vi "8HP_Standard_EnFlo_Specific.vi"(2 "Datalog file path (full)":path, 3 "COM port":refnum<visa-resource-name>, 4 "Log data stream":bool, 5 "Set data rate (Hz)":u8(ring)=14 items=["1", "2", "4", "5", "8", "10", "16", "20", "25", "32", "40", "50", "64", "80", "100", "125", "160", "200", "250", "320", "400", "500", "625", "800", "1000"], 6 "N samples":u32=1000, 7 "Command":T2="s") -> (0 "Error":errorcluster, 1 "All samples out":sgl[][](array[numeric]))   [LabVIEW 2020]
uses:
  ctls/8HP_Cmd (USB).ctl
  Globals/Meas_global.vi
panel:
  in  "Main":T1(tab)
  out "Serial number":sgl
  out "Subsystems ok":bool[](array[boolean])
  out "Pressure sensor values in range":bool[](array[boolean])
  out "Pressure sensor temperatures in range":bool[](array[boolean])
  out "Pressure sensor EEPROM checksums ok":bool[](array[boolean])
  out "P_raw_Azero":sgl[](array[numeric])
  out "n":u16
  out "Auto zero progBar":u16(slide) caption="Collecting samples, please maintain dP = 0" scale=0.0..1000.0
  in  "EEPROM array 2":u16[](array[numeric])
  in  "EEPROM array":sgl[](array[numeric])
  out "Chk ok":bool
  out "EEPROM Checksum":u8 format="%02x"
  out "received":bool
  out "Returned data rate (Hz)":u16
  out "sent":bool
  out "frm err":u32
  out "chk err":u32
  in  "Stop Data":bool
  out "Relative humidity (%)":sgl
  out "Env. sensor die temperature (deg C)":sgl
  out "External thermistor 0 temperature (deg C)":sgl
  out "Atmospheric pressure (mbar)":sgl
  out "Checksum ok":bool
  out "Gyration vector (deg / s)":sgl[](array[numeric])
  out "Acceleration vector (g)":sgl[](array[numeric])
  out "Pressures":sgl[][](graph)
  out "Stream enabled":bool
  out "External thermistor 1 temperature (deg C)":sgl
  # "Paul Nathan 07/2023"
  # "Output array order:\nP0 (Pa)\n  |\nP7 (Pa)\nT0 (deg C)\nT1 (deg C)\nP_atmos (mbar)\nT_env (deg C)\nRH (%)\nax (g)\nay (g)\naz (g)\nwx (deg / s)\nwy (deg / s)\nwz (deg / s)"
  # "Environmental sensor present"
  # "Inertial sensor present"
  # "Accelerometer self test pass"
  # "Gyroscope self test pass"
  # "External thermistor 0 value in range"
  # "External thermistor 1 value in range"
  # "MCU EEPROM checksum ok"
  # "Pressure sensor 0 value in range"
  # "Pressure sensor 1 value in range"
  # "Pressure sensor 2 value in range"
  # "Pressure sensor 3 value in range"
  # "Pressure sensor 4 value in range"
  # "Pressure sensor 5 value in range"
  # "Pressure sensor 6 value in range"
  # "Pressure sensor 7 value in range"
  # "Pressure sensor 0 temperature in range"
  # "Pressure sensor 1 temperature in range"
  # "Pressure sensor 2 temperature in range"
  # "Pressure sensor 3 temperature in range"
  # "Pressure sensor 4 temperature in range"
  # "Pressure sensor 5 temperature in range"
  # "Pressure sensor 6 temperature in range"
  # "Pressure sensor 7 temperature in range"
  # "Pressure sensor 0 EEPROM checksum okay"
  # "Pressure sensor 1 EEPROM checksum okay"
  # "Pressure sensor 2 EEPROM checksum okay"
  # "Pressure sensor 3 EEPROM checksum okay"
  # "Pressure sensor 4 EEPROM checksum okay"
  # "Pressure sensor 5 EEPROM checksum okay"
  # "Pressure sensor 6 EEPROM checksum okay"
  # "Pressure sensor 7 EEPROM checksum okay"
  # "of 1000"
  # "P0 raw auto-zero"
  # "P1 raw auto-zero"
  # "P2 raw auto-zero"
  # "P3 raw auto-zero"
  # "P4 raw auto-zero"
  # "P5 raw auto-zero"
  # "P6 raw auto-zero"
  # "P7 raw auto-zero"
  # "Power-up defaults"
  # "Data rate (Hz)"
  # "TTL streaming"
  # "USB streaming"
  # "TTL stream contains full data"
  # "Accelerometer range mode"
  # "Gyroscope range mode"
  # "IMU rate mode"
  # "P0 raw auto-zero"
  # "P1 raw auto-zero"
  # "P2 raw auto-zero"
  # "P3 raw auto-zero"
  # "P4 raw auto-zero"
  # "P5 raw auto-zero"
  # "P6 raw auto-zero"
  # "P7 raw auto-zero"
  # "Atmospheric pressure offset (Pa)"
  # "External thermistor 0 temperature offset (deg C)"
  # "External thermistor 1 temperature offset (deg C)"
  # "Serial number"
  # "Baud rate (bps)"
  # "Accelerometer vector magnitude scale factor"
  # "Gyroscope x component offset (deg / s)"
  # "Gyroscope y component offset (deg / s)"
  # "Gyroscope z component offset (deg / s)"
  # "w_x"
  # "w_y"
  # "w_z"
  # "a_x"
  # "a_y"
  # "a_z"
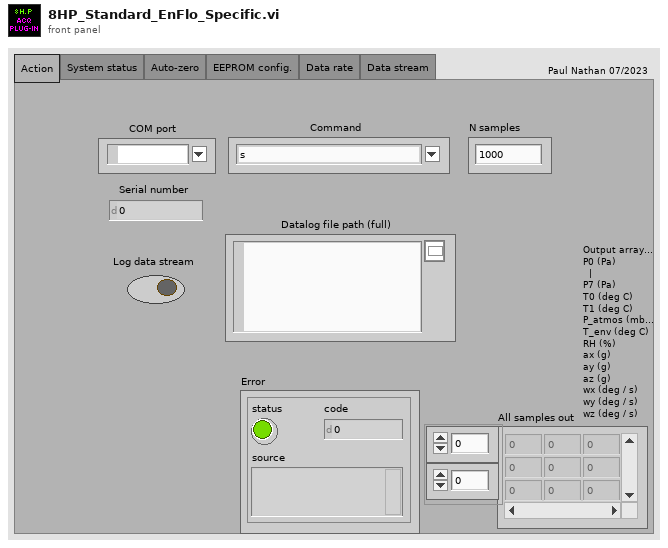
[diagram p1: front panel]
types:
  T1 = enum32{"Action", "System status", "Auto-zero", "EEPROM config.", "Data rate", "Data stream"}
  T2 = typedef "8HP_Cmd (USB).ctl" = string
  T3 = enum16{"open", "replace", "create", "open or create", "replace or create", "replace or create with confirmation"}
  T4 = typedef "Rendezvous RefNum" = refnum<k1>
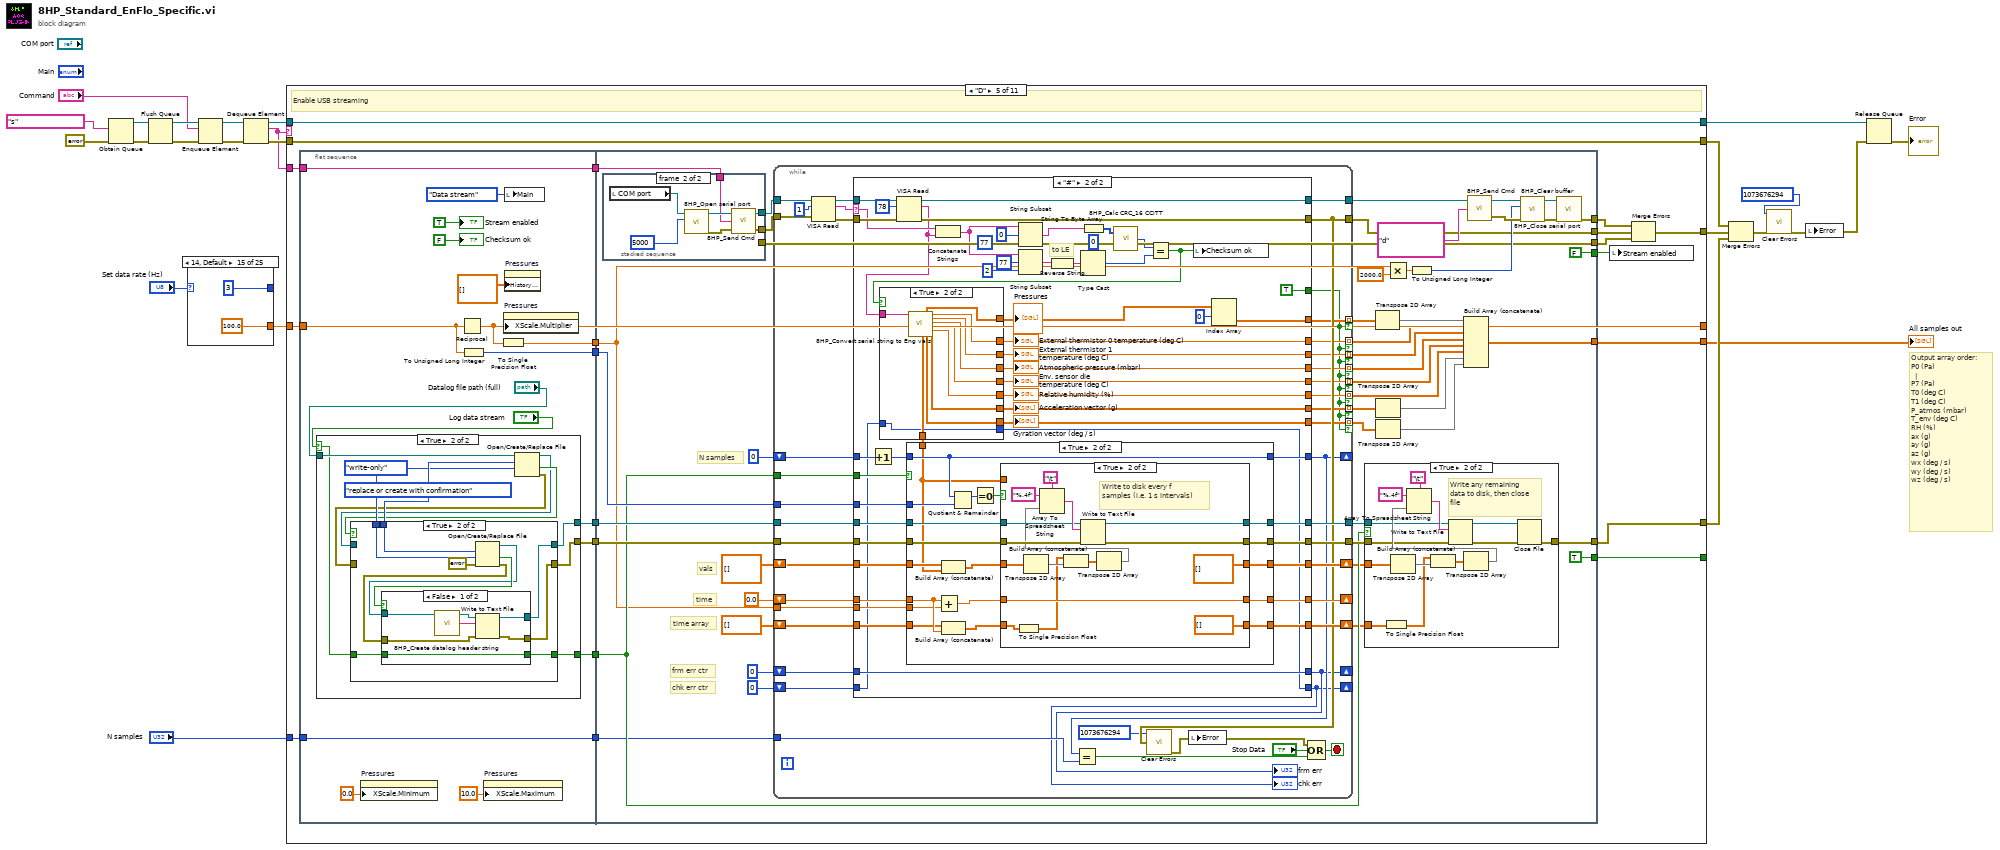
[diagram p0: block diagram]
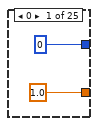
[diagram p2: hidden frame]
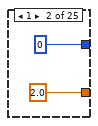
[diagram p3: hidden frame]
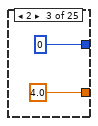
[diagram p4: hidden frame]
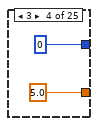
[diagram p5: hidden frame]
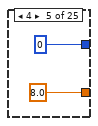
[diagram p6: hidden frame]
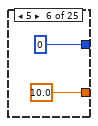
[diagram p7: hidden frame]
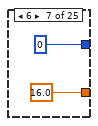
[diagram p8: hidden frame]
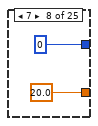
[diagram p9: hidden frame]
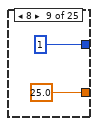
[diagram p10: hidden frame]
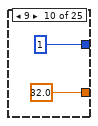
[diagram p11: hidden frame]
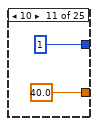
[diagram p12: hidden frame]
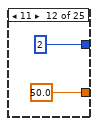
[diagram p13: hidden frame]
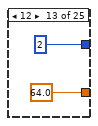
[diagram p14: hidden frame]
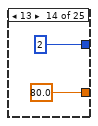
[diagram p15: hidden frame]
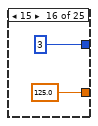
[diagram p16: hidden frame]
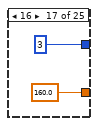
[diagram p17: hidden frame]
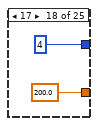
[diagram p18: hidden frame]
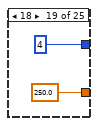
[diagram p19: hidden frame]
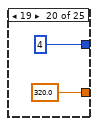
[diagram p20: hidden frame]
diagram:
  # "Output array order:\nP0 (Pa)\n  |\nP7 (Pa)\nT0 (deg C)\nT1 (deg C)\nP_atmos (mbar)\nT_env (deg C)\nRH (%)\nax (g)\nay (g)\naz (g)\nwx (deg / s)\nwy (deg / s)\nwz (deg / s)"
  n1 = Obtain Queue(element data type=T2 "s" ("Combo Box"), error in (no error)=errorcluster {"status"=FALSE, "code"=0, "source"=""}) -> (queue out=w22:refnum<queue>, error out=w23:errorcluster)  [unwired: 3 in, 1 out]
  n2 = Flush Queue(queue=w22, error in (no error)=w23) -> (queue out=w17:refnum<queue>, error out=w16:errorcluster)  [unwired: 1 out]
  n3 = case shown="14, Default" "Set data rate (Hz)" {
    tunnel: [1.0 2.0 4.0 5.0 8.0 10.0 16.0 20.0 25.0 32.0 40.0 50.0 64.0 80.0 100.0 125.0 160.0 200.0 250.0 320.0 400.0 500.0 625.0 800.0 1000.0] -> w4
    tunnel: [u8 0 u8 0 u8 0 u8 0 u8 0 u8 0 u8 0 u8 0 u8 1 u8 1 u8 1 u8 2 u8 2 u8 2 u8 3 u8 3 u8 3 u8 4 u8 4 u8 4 u8 5 u8 5 u8 6 u8 6 u8 6] -> _
    frame 0 {
    }
    frame 1 {
    }
    frame 2 {
    }
    frame 3 {
    }
    frame 4 {
    }
    frame 5 {
    }
    frame 6 {
    }
    frame 7 {
    }
    frame 8 {
    }
    frame 9 {
    }
    frame 10 {
    }
    frame 11 {
    }
    frame 12 {
    }
    frame 13 {
    }
    frame 14, Default {
    }
    frame 15 {
    }
    frame 16 {
    }
    frame 17 {
    }
    frame 18 {
    }
    frame 19 {
    }
    frame 20 {
    }
    frame 21 {
    }
    frame 22 {
    }
    frame 23 {
    }
    frame 24 {
    }
  }
  n4 = Enqueue Element(queue=w17, element="Command", error in (no error)=w16) -> (queue out=w19:refnum<queue>, error out=w18:errorcluster)  [unwired: 1 in, 1 out]
  n5 = Dequeue Element(queue=w19, error in (no error)=w18) -> (queue out=w14:refnum<queue>, element=w12:T2, error out=w13:errorcluster)  [unwired: 1 in, 1 out]
  n6 = case shown="\"D\"" w12 {
    tunnel: [w81 w122 w161 w237 w315 w618 w644 w727 w767 FALSE FALSE] -> _
    tunnel: w14 -> [w80 w121 w160 w236 w314 w620 w646 w729 w766 w791 w796]
    tunnel: [w80 w121 w160 w236 w314 w620 w646 w729 w766 w791 w796] -> w6
    tunnel: w13 -> [w79 w120 w159 w235 w313 w619 w647 w730 w765 w790 w795]
    tunnel: [w79 w120 w159 w235 w313 w619 w647 w730 w765 w790 w795] -> w11
    tunnel: w12 -> [w78 w119 w158 w234 w312 w622 w652 w735 w764 _ _]
    tunnel: [w76 w117 w156 w231 w298 w621 w645 w728 w762 errorcluster {"status"=FALSE, "code"=0, "source"=""} ("Error out") errorcluster {"status"=FALSE, "code"=0, "source"=""} ("Error out")] -> w10
    tunnel: [_ _ _ _ w310 _ _ _ _ _ _] -> w9
    tunnel: w4 -> [w75 w116 w155 w230 w303 w616 _ _ w761 w787 w792]
    tunnel: [w75 w116 w155 w230 w303 w616 w648 w731 w761 w787 w792] -> _
    tunnel: [_ _ _ _ w302 _ _ _ _ _ _] -> w2
    tunnel: "N samples" -> [_ _ _ _ w296 _ _ _ _ _ _]
    frame "S", "s" {
      # "Perform self-test and retrieve status bytes, Retrieve status bytes"
      n7 = flat-sequence {
        tunnel: w78 -> [w84]
        tunnel: [w84] -> w77
        tunnel: [TRUE] -> w81
        tunnel: w77 -> [w90]
        tunnel: [w85] -> w76
        frame #0 {
          w83 = bool[] [] ("Pressure sensor EEPROM checksums ok")
          n8 = local write "Main"(T1."System status" ("Main")) -> ()
          "Pressure sensor EEPROM checksums ok" <- w83
          "Pressure sensor temperatures in range" <- w83
          "Pressure sensor values in range" <- w83
          "Subsystems ok" <- w83
        }
        frame #1 {
          w95 = 1 ("length (rest)")
          w103 = u8 0 ("byte count")
          n9 = local read "COM port"() -> (w91:refnum<visa-resource-name>)
          n10 = call "8HP_Open serial port.vi"("timeout (ms)"=u32 5000, "VISA resource name"=w91) -> ("Error out"=w113:errorcluster, "VISA resource name out"=w114:refnum<visa-resource-name>)  [unwired: 8 in]
          n11 = call "8HP_Send Cmd.vi"("Error In"=w113, "Operation"=w90, "Port"=w114) -> ("Error Out"=w111:errorcluster, "Port out"=w112:refnum<visa-resource-name>)  [unwired: 1 in]
          n12 = VISA Read(VISA resource name=w112, byte count=u32 4, error in (no error)=w111) -> (VISA resource name out=w109:refnum<visa-resource-name>, read buffer=w98:string, error out=w108:errorcluster)  [unwired: 1 out]
          n13 = call "8HP_Close serial port.vi"("Error in"=w108, "VISA resource name"=w109) -> ("Error out"=w85:errorcluster)  [unwired: 9 in]
          n14 = String Subset(string=w98, offset (0)=0, length (rest)=w95) -> (substring=w107:string)
          n15 = String Subset(string=w98, offset (0)=1, length (rest)=w95) -> (substring=w106:string)
          n16 = String Subset(string=w98, offset (0)=2 ("length (rest)"), length (rest)=w95) -> (substring=w105:string)
          n17 = String Subset(string=w98, offset (0)=3, length (rest)=w95) -> (substring=w104:string)
          n18 = Type Cast(type=w103, x=w107) -> (*(type *) &x=w102:u8)
          n19 = Type Cast(type=w103, x=w106) -> (*(type *) &x=w101:u8)
          n20 = Type Cast(type=w103, x=w105) -> (*(type *) &x=w100:u8)
          n21 = Type Cast(type=w103, x=w104) -> (*(type *) &x=w99:u8)
          n22 = Number To Boolean Array(number=w102) -> (Boolean array=w89:bool[])
          n23 = Number To Boolean Array(number=w101) -> (Boolean array=w88:bool[])
          n24 = Number To Boolean Array(number=w100) -> (Boolean array=w87:bool[])
          n25 = Number To Boolean Array(number=w99) -> (Boolean array=w86:bool[])
          n26 = local write "Pressure sensor EEPROM checksums ok"(w89) -> ()
          n27 = local write "Pressure sensor temperatures in range"(w88) -> ()
          n28 = local write "Pressure sensor values in range"(w87) -> ()
          n29 = local write "Subsystems ok"(w86) -> ()
        }
      }
    }
    frame "Z", "z" {
      # "Perform permanent auto-zero (write values to EEPROM), Perform temporary auto-zero"
      n30 = flat-sequence {
        tunnel: w119 -> [w126]
        tunnel: [w126] -> w118
        tunnel: [TRUE] -> w122
        tunnel: w118 -> [w133]
        tunnel: [w129] -> w117
        frame #0 {
          n31 = local write "Main"(T1."Auto-zero" ("Main")) -> ()
          "P_raw_Azero" <- sgl[] [] ("P_raw_Azero")
          "Auto zero progBar" <- u16 0 ("Collecting samples, please maintain dP = 0")
        }
        frame #1 {
          n32 = local read "COM port"() -> (w134:refnum<visa-resource-name>)
          n33 = call "8HP_Open serial port.vi"("timeout (ms)"=u32 16000, "VISA resource name"=w134) -> ("Error out"=w141:errorcluster, "VISA resource name out"=w142:refnum<visa-resource-name>)  [unwired: 8 in]
          n34 = call "8HP_Send Cmd.vi"("Error In"=w141, "Operation"=w133, "Port"=w142) -> ("Error Out"=w139:errorcluster, "Port out"=w140:refnum<visa-resource-name>)  [unwired: 1 in]
          n35 = VISA Read(VISA resource name=w140, byte count=u32 32, error in (no error)=w139) -> (VISA resource name out=w137:refnum<visa-resource-name>, read buffer=w130:string, error out=w136:errorcluster)  [unwired: 1 out]
          n36 = for {
            N: 1000 -> [_]
            shift-right: [w144] -> _
            shift-left: u16 0 -> [w145]
            n37 = Increment(x=w145) -> (x+1=w144:u16)
            "n" <- w144
            n38 = Wait (ms)(milliseconds to wait=u32 10) -> ()  [unwired: 1 out]
            n39 = local write "Auto zero progBar"(w144) -> ()
          }
          n40 = for {
            N: 8 -> [_]
            tunnel: [w148] -> w132 mode=indexing
            tunnel: w130 -> [w147]
            i -> [w154]
            w152 = 4 ("x")
            # "to BE"
            n41 = Multiply(x=w152, y=w154) -> (x*y=w153:i32)
            n42 = String Subset(string=w147, offset (0)=w153, length (rest)=w152) -> (substring=w151:string)
            n43 = Reverse String(1:w151) -> (0:w150:string)
            n44 = Type Cast(type=sgl 0.0 ("byte count"), x=w150) -> (*(type *) &x=w148:sgl)
          }
          n45 = call "8HP_Close serial port.vi"("Error in"=w136, "VISA resource name"=w137) -> ("Error out"=w129:errorcluster)  [unwired: 9 in]
          n46 = local write "P_raw_Azero"(w132) -> ()
        }
      }
    }
    frame "R" {
      # "Read all EEPROM values"
      n47 = flat-sequence {
        tunnel: w158 -> [w165]
        tunnel: [w165] -> w157
        tunnel: [TRUE] -> w161
        tunnel: w157 -> [w200]
        tunnel: [w189] -> w156
        frame #0 {
          n48 = local write "EEPROM array"(sgl[] [] ("EEPROM array")) -> ()
          n49 = local write "EEPROM array 2"(u16[] [] ("EEPROM array 2")) -> ()
          n50 = local write "Main"(T1."EEPROM config." ("Main")) -> ()
        }
        frame #1 {
          # "to BE"
          n51 = local read "COM port"() -> (w201:refnum<visa-resource-name>)
          n52 = call "8HP_Open serial port.vi"("timeout (ms)"=u32 5000, "VISA resource name"=w201) -> ("Error out"=w208:errorcluster, "VISA resource name out"=w209:refnum<visa-resource-name>)  [unwired: 8 in]
          n53 = call "8HP_Send Cmd.vi"("Error In"=w208, "Operation"=w200, "Port"=w209) -> ("Error Out"=w206:errorcluster, "Port out"=w207:refnum<visa-resource-name>)  [unwired: 1 in]
          n54 = VISA Read(VISA resource name=w207, byte count=u32 78, error in (no error)=w206) -> (VISA resource name out=w204:refnum<visa-resource-name>, read buffer=w172:string, error out=w203:errorcluster)  [unwired: 1 out]
          n55 = String To Byte Array(string=w172) -> (unsigned byte array=w192:u8[])
          n56 = call "8HP_Close serial port.vi"("Error in"=w203, "VISA resource name"=w204) -> ("Error out"=w189:errorcluster)  [unwired: 9 in]
          n57 = String Subset(string=w172, offset (0)=0, length (rest)=56 ("length (rest)")) -> (substring=w187:string)
          n58 = String Subset(string=w172, offset (0)=64, length (rest)=12 ("length (rest)")) -> (substring=w182:string)
          n59 = String Subset(string=w172, offset (0)=56, length (rest)=2 ("length (rest)")) -> (substring=w171:string)
          n60 = String Subset(string=w172, offset (0)=58, length (rest)=6 ("length (rest)")) -> (substring=w166:string)
          n61 = Array Size(array=w192) -> (size(s)=w194:i32)
          n62 = Decrement(x=w194) -> (x-1=w193:i32)
          n63 = for {
            N: 14 -> [_]
            tunnel: [w222] -> w181 mode=indexing
            tunnel: w187 -> [w221]
            i -> [w226]
            w224 = 4 ("x")
            # "to BE"
            n64 = Multiply(x=w224, y=w226) -> (x*y=w225:i32)
            n65 = String Subset(string=w221, offset (0)=w225, length (rest)=w224) -> (substring=w220:string)
            n66 = Reverse String(1:w220) -> (0:w219:string)
            n67 = Type Cast(type=sgl 0.0 ("byte count"), x=w219) -> (*(type *) &x=w222:sgl)
          }
          n68 = for {
            N: 3 -> [_]
            tunnel: [w214] -> w180 mode=indexing
            tunnel: w182 -> [w213]
            i -> [w218]
            w216 = 4 ("x")
            # "to BE"
            n69 = Multiply(x=w216, y=w218) -> (x*y=w217:i32)
            n70 = String Subset(string=w213, offset (0)=w217, length (rest)=w216) -> (substring=w212:string)
            n71 = Reverse String(1:w212) -> (0:w211:string)
            n72 = Type Cast(type=sgl 0.0 ("byte count"), x=w211) -> (*(type *) &x=w214:sgl)
          }
          n73 = Index Array(array=w192, index=77) -> (element=w196:u8)
          n74 = Array Subset(array=w192, index=0, length=w193) -> (w190:u8[])
          n75 = Reverse String(1:w171) -> (0:w178:string)
          n76 = Add Array Elements(numeric array=w190) -> (sum=w191:u8)
          n77 = Type Cast(type=u16 0 ("byte count"), x=w178) -> (*(type *) &x=w170:u16)
          n78 = String To Byte Array(string=w166) -> (unsigned byte array=w169:u8[])
          n79 = To Unsigned Word Integer(number=w169) -> (unsigned 16bit integer=w167:u16[])
          n80 = Equal?(x=w196, y=w191) -> (x = y?=w198:bool)
          n81 = Build Array (concatenate)(w181, w180) -> (w179:sgl[])
          n82 = Build Array (concatenate)(w170, w167) -> (w168:u16[])
          n83 = local write "EEPROM array"(w179) -> ()
          n84 = local write "EEPROM array 2"(w168) -> ()
          n85 = local write "EEPROM Checksum"(w196) -> ()
          n86 = local write "Chk ok"(w198) -> ()
        }
      }
    }
    frame "W" {
      # "Write all EEPROM values (including new checksum)"
      n87 = flat-sequence {
        tunnel: w234 -> [w250]
        tunnel: [w250] -> w233
        tunnel: [w244] -> w232
        tunnel: [w243] -> w229
        tunnel: [w239] -> w228
        tunnel: [w240] -> w227
        tunnel: [TRUE] -> w237
        tunnel: w233 -> [w278]
        tunnel: w232 -> [w272]
        tunnel: [w270] -> w231
        tunnel: w229 -> [w259]
        tunnel: w228 -> [w256]
        tunnel: w227 -> [w254]
        frame #0 {
          n88 = local write "Main"(T1."EEPROM config." ("Main")) -> ()
          n89 = Split 1D Array(array="EEPROM array", index=14) -> (first subarray=w244:sgl[], second subarray=w243:sgl[])
          n90 = Split 1D Array(array="EEPROM array 2", index=1) -> (first subarray=w242:u16[], second subarray=w241:u16[])
          n91 = Index Array(array=w242, index=0) -> (element=w239:u16)
          n92 = To Unsigned Byte Integer(number=w241) -> (unsigned 8bit integer=w240:u8[])
        }
        frame #1 {
          # "to LE"
          n93 = local read "COM port"() -> (w279:refnum<visa-resource-name>)
          n94 = for {
            N: 14 -> [_]
            tunnel: w272 -> [w292] mode=indexing
            shift-right: [w293] -> w265
            shift-left: "" -> [w294]
            # "to LE"
            n95 = Type Cast(type="", x=w292) -> (*(type *) &x=w291:string)
            n96 = Reverse String(1:w291) -> (0:w290:string)
            n97 = Concatenate Strings(w294, w290) -> (w293:string)
          }
          n98 = for {
            N: 3 -> [_]
            tunnel: w259 -> [w286] mode=indexing
            shift-right: [w287] -> w252
            shift-left: "" -> [w288]
            # "to LE"
            n99 = Type Cast(type="", x=w286) -> (*(type *) &x=w285:string)
            n100 = Reverse String(1:w285) -> (0:w284:string)
            n101 = Concatenate Strings(w288, w284) -> (w287:string)
          }
          n102 = Type Cast(type="", x=w256) -> (*(type *) &x=w258:string)
          n103 = Reverse String(1:w258) -> (0:w255:string)
          n104 = Byte Array To String(unsigned byte array=w254) -> (string=w251:string)
          n105 = call "8HP_Open serial port.vi"("timeout (ms)"=u32 5000, "VISA resource name"=w279) -> ("Error out"=w281:errorcluster, "VISA resource name out"=w282:refnum<visa-resource-name>)  [unwired: 8 in]
          n106 = Type Cast(type="", x=u8 0) -> (*(type *) &x=w253:string)
          n107 = Concatenate Strings(w265, w255, w251, w252, w253) -> (w262:string)
          n108 = String To Byte Array(string=w262) -> (unsigned byte array=w266:u8[])
          n109 = Add Array Elements(numeric array=w266) -> (sum=w271:u8)
          "EEPROM Checksum" <- w271
          n110 = Type Cast(type="", x=w271) -> (*(type *) &x=w274:string)
          n111 = Concatenate Strings(w262, w274) -> (w269:string)
          n112 = call "8HP_Send Cmd + Data.vi"("Error In"=w281, "Data"=w269, "Operation"=w278, "Port"=w282) -> ("Error Out"=w267:errorcluster, "Port out"=w268:refnum<visa-resource-name>)  [unwired: 1 in]
          n113 = call "8HP_Close serial port.vi"("Error in"=w267, "VISA resource name"=w268) -> ("Error out"=w270:errorcluster)  [unwired: 9 in]
          "Chk ok" <- TRUE ("Chk ok")
        }
      }
    }
    frame "D" {
      # "Enable USB streaming"
      n114 = flat-sequence {
        tunnel: w312 -> [w332]
        tunnel: [w332] -> w311
        tunnel: [w329] -> w309
        tunnel: [w328] -> w308
        tunnel: [w327] -> w307
        tunnel: w303 -> [w318]
        tunnel: [w325] -> w306
        tunnel: [w321] -> w305
        tunnel: [w319] -> w297
        tunnel: w296 -> [w319]
        tunnel: [TRUE] -> w315
        tunnel: w311 -> [w388]
        tunnel: [w415] -> w300
        tunnel: [w414] -> w310
        tunnel: w309 -> [w411]
        tunnel: w308 -> [w410]
        tunnel: w307 -> [w412]
        tunnel: w306 -> [w394]
        tunnel: w305 -> [w404]
        tunnel: [FALSE] -> w304
        tunnel: [w384] -> w302
        tunnel: [w375] -> w299
        tunnel: [w374] -> w301
        tunnel: w297 -> [w373]
        frame #0 {
          n115 = case shown="True" "Log data stream" {
            selector: "Log data stream" -> [w333 w336]
            tunnel: "Datalog file path (full)" -> [_ w345]
            tunnel: [refnum<file> refnum ("refnum out") w342] -> w329
            tunnel: [errorcluster {"status"=FALSE, "code"=0, "source"=""} ("error out") w341] -> w328
            tunnel: [w333 w337] -> w321
            frame False {
            }
            frame True {
              w343 = enum16{"read/write", "read-only", "write-only"}."write-only" ("access (0:read/write)")
              w344 = T3."replace or create with confirmation" ("operation (0:open)")
              n116 = Open/Create/Replace File(file path (use dialog)=w345, operation (0:open)=w344, access (0:read/write)=w343) -> (refnum out=w338:refnum<file>, cancelled=w340:bool, error out=w339:errorcluster)  [unwired: 3 in]
              n117 = case shown="True" w340 {
                tunnel: w344 -> [_ w361]
                tunnel: w343 -> [_ w360]
                tunnel: w339 -> [w349 _]
                tunnel: [w347 w355] -> w342
                tunnel: [w348 w356] -> w341
                tunnel: w338 -> [w350 _]
                tunnel: [w346 w353] -> w337
                tunnel: w336 -> [w346 w352]
                frame False {
                  n118 = call "8HP_Create datalog header string.vi"() -> ("Datalog header string"=w351:string)  [unwired: 1 in]
                  n119 = Write to Text File(file (use dialog)=w350, text=w351, error in=w349) -> (refnum out=w347:refnum<file>, error out=w348:errorcluster)  [unwired: 1 in, 1 out]
                }
                frame True {
                  n120 = Open/Create/Replace File(error in=errorcluster {"status"=FALSE, "code"=0, "source"=""}, operation (0:open)=w361, access (0:read/write)=w360) -> (refnum out=w358:refnum<file>, cancelled=w359:bool, error out=w357:errorcluster)  [unwired: 3 in]
                  n121 = case shown="False" w359 {
                    tunnel: w358 -> [w366 _]
                    tunnel: w357 -> [w365 _]
                    tunnel: [w364 errorcluster {"status"=FALSE, "code"=0, "source"=""} ("error out")] -> w356
                    tunnel: [w363 refnum<file> refnum ("t")] -> w355
                    tunnel: [w362 w368] -> w353
                    tunnel: w352 -> [w362 _]
                    frame False {
                      n122 = call "8HP_Create datalog header string.vi"() -> ("Datalog header string"=w367:string)  [unwired: 1 in]
                      n123 = Write to Text File(file (use dialog)=w366, text=w367, error in=w365) -> (refnum out=w363:refnum<file>, error out=w364:errorcluster)  [unwired: 1 in, 1 out]
                    }
                    frame True {
                      w368 = FALSE ("Log data stream")
                      n124 = local write "Log data stream"(w368) -> ()
                    }
                  }
                }
              }
            }
          }
          n125 = property on="Pressures" class="WFChart (strict)"("XScale.Minimum"=0.0 ("X Scale.Range:Minimum")) -> ()  [unwired: 2 in, 2 out]
          n126 = Reciprocal(x=w318) -> (1/x=w326:dbl)
          n127 = To Unsigned Long Integer(number=w318) -> (unsigned 32bit integer=w327:u32)
          n128 = property on="Pressures" class="WFChart (strict)"("XScale.Maximum"=10.0 ("X Scale.Range:Minimum")) -> ()  [unwired: 2 in, 2 out]
          n129 = To Single Precision Float(number=w326) -> (single precision float=w325:sgl)
          n130 = property on="Pressures" class="WFChart (strict)"("XScale.Multiplier"=w326) -> ()  [unwired: 2 in, 2 out]
          n131 = local write "Main"(T1."Data stream" ("Main")) -> ()
          n132 = property on="Pressures" class="WFChart (strict)"("History Data"=sgl[][] []) -> ()  [unwired: 2 in, 2 out]
          "Checksum ok" <- FALSE ("Checksum ok")
          "Stream enabled" <- TRUE ("Stream enabled")
        }
        frame #1 {
          # "chk err ctr"
          # "frm err ctr"
          # "N samples"
          # "vals"
          # "time"
          # "time array"
          n133 = stacked-sequence {
            tunnel: [_ w424] -> w403
            tunnel: [_ w422] -> w402
            tunnel: w388 -> [_ w420]
            tunnel: [w418 _] -> w375
            frame #0 {
              # "Wait here until all acq. devs. are ready."
              n134 = global read "Meas_global.vi" "Acquisition Rendezvous"() -> (w419:T4)
              n135 = call <vilib>:"Wait at Rendezvous.vi"("ms timeout (-1)"=60000, "rendezvous"=w419) -> ("error out"=w418:errorcluster)  [unwired: 3 in, 2 out]
            }
            frame #1 {
              n136 = local read "COM port"() -> (w426:refnum<visa-resource-name>)
              n137 = call "8HP_Open serial port.vi"("timeout (ms)"=u32 5000, "VISA resource name"=w426) -> ("Error out"=w423:errorcluster, "VISA resource name out"=w425:refnum<visa-resource-name>)  [unwired: 8 in]
              n138 = call "8HP_Send Cmd.vi"("Error In"=w423, "Operation"=w420, "Port"=w425) -> ("Error Out"=w422:errorcluster, "Port out"=w424:refnum<visa-resource-name>)  [unwired: 1 in]
            }
          }
          n139 = while {
            tunnel: [w460] -> w374
            tunnel: w403 -> [w462]
            tunnel: [w479] -> w401
            shift-right: [w445] -> _
            shift-left: u32 0 -> [w476]
            tunnel: w412 -> [w475]
            tunnel: w411 -> [w474]
            tunnel: w410 -> [w473]
            tunnel: [w472] -> w409
            tunnel: [w471] -> w408
            shift-right: [w470] -> w391
            shift-left: sgl[][] [] -> [w469]
            shift-right: [w466] -> _
            shift-left: sgl 0.0 ("Numeric") -> [w468]
            tunnel: w394 -> [w467]
            shift-right: [w464] -> w390
            shift-left: sgl[] [] -> [w465]
            tunnel: w404 -> [w463]
            tunnel: w402 -> [w461]
            tunnel: [w457] -> w383 mode=indexing if=w449
            tunnel: [w456] -> w382 mode=indexing if=w449
            tunnel: [w455] -> w381 mode=indexing if=w449
            tunnel: [w454] -> w380 mode=indexing if=w449
            tunnel: [w453] -> w379 mode=indexing if=w449
            tunnel: [w452] -> w376 mode=indexing if=w449
            tunnel: [w451] -> w377 mode=indexing if=w449
            tunnel: [w450] -> w378 mode=indexing if=w449
            tunnel: w373 -> [w447]
            shift-right: [w443] -> _
            shift-left: u32 0 -> [w448]
            shift-right: [w442] -> _
            shift-left: u32 0 -> [w444]
            stop <- w477 stop-if-true
            n140 = VISA Read(VISA resource name=w462, byte count=u32 1, error in (no error)=w461) -> (VISA resource name out=w481:refnum<visa-resource-name>, read buffer=w482:string, error out=w480:errorcluster)  [unwired: 1 out]
            n141 = case shown="\"#\"" w482 {
              selector: w482 -> [_ w541]
              tunnel: w481 -> [w494 w545]
              tunnel: [w495 w543] -> w460
              tunnel: w480 -> [w495 w546]
              tunnel: [w494 w544] -> w479
              tunnel: w476 -> [w493 w500]
              tunnel: [w493 w539] -> w445
              tunnel: w475 -> [_ w538]
              tunnel: w474 -> [w492 w537]
              tunnel: w473 -> [w491 w536]
              tunnel: [w491 w535] -> w472
              tunnel: [w492 w534] -> w471
              tunnel: [w490 w533] -> w470
              tunnel: w469 -> [w490 w532]
              tunnel: w468 -> [w489 w531]
              tunnel: w467 -> [_ w530]
              tunnel: [w489 w529] -> w466
              tunnel: w465 -> [w488 w528]
              tunnel: [w488 w527] -> w464
              tunnel: w463 -> [_ w526]
              tunnel: [_ w525] -> w457
              tunnel: [FALSE TRUE] -> w449
              tunnel: [_ w516] -> w456
              tunnel: [_ w515] -> w455
              tunnel: [_ w514] -> w454
              tunnel: [_ w520] -> w453
              tunnel: [_ w519] -> w452
              tunnel: [_ w518] -> w451
              tunnel: [_ w517] -> w450
              tunnel: w448 -> [w486 w498]
              tunnel: [w485 w498] -> w443
              tunnel: w444 -> [w484 w497]
              tunnel: [w484 w496] -> w442
              frame Default {
                # "Frame error"
                n142 = Increment(x=w486) -> (x+1=w485:u32)
              }
              frame "#" {
                # "to LE"
                n143 = Increment(x=w500) -> (x+1=w499:u32)
                n144 = VISA Read(VISA resource name=w545, byte count=u32 78, error in (no error)=w546) -> (VISA resource name out=w544:refnum<visa-resource-name>, read buffer=w540:string, error out=w543:errorcluster)  [unwired: 1 out]
                n145 = Concatenate Strings(w541, w540) -> (w504:string)
                n146 = String Subset(string=w504, offset (0)=0, length (rest)=77 ("length (rest)")) -> (substring=w513:string)
                n147 = String Subset(string=w504, offset (0)=77, length (rest)=2 ("length (rest)")) -> (substring=w508:string)
                n148 = Reverse String(1:w508) -> (0:w509:string)
                n149 = String To Byte Array(string=w513) -> (unsigned byte array=w503:u8[])
                n150 = Type Cast(type=u16 0 ("length (rest)"), x=w509) -> (*(type *) &x=w510:u16)
                n151 = call "8HP_Calc CRC_16 CCITT.vi"("Data bytes"=w503) -> ("CRC_16-CCITT"=w502:u16)  [unwired: 1 in]
                n152 = Equal?(x=w502, y=w510) -> (x = y?=w501:bool)
                n153 = case shown="True" w501 {
                  tunnel: w540 -> [_ w569]
                  tunnel: [w558 w568] -> w516
                  tunnel: [w558 w567] -> w515
                  tunnel: [w558 w566] -> w520
                  tunnel: [w558 w565] -> w519
                  tunnel: [w556 w564] -> w518
                  tunnel: [w556 w563] -> w517
                  tunnel: [w553 w562] -> w524
                  tunnel: [w558 w561] -> w514
                  tunnel: [w549 w560] -> w522
                  tunnel: w497 -> [w548 w559]
                  tunnel: [w547 w559] -> w496
                  frame False {
                    (unwired) 3 ("dimension size")
                    w558 = sgl nan ("Atmospheric pressure (mbar)")
                    n154 = Increment(x=w548) -> (x+1=w547:u32)
                    n155 = Initialize Array(sgl nan ("element"), 8 ("dimension size")) -> (w552:sgl[])
                    n156 = Initialize Array(sgl nan ("element")) -> (w556:sgl[])  [unwired: 1 in]
                    n157 = Initialize Array(sgl nan ("element"), 19 ("dimension size")) -> (w553:sgl[])
                    n158 = Build Array(w552) -> (w549:sgl[][])
                  }
                  frame True {
                    n159 = call "8HP_Convert serial string to Eng vals.vi"("Serial buffer string (excluding FrameChar)"=w569) -> ("All vals"=w562:sgl[], "Pressures"=w560:sgl[][], "Gyration vector (deg / s)"=w563:sgl[], "External thermistor 0 temperature (°C)"=w568:sgl, "External thermistor 1 temperature (°C)"=w567:sgl, "Atmospheric pressure (mbar)"=w561:sgl, "Env. sensor die temperature (°C)"=w566:sgl, "Relative humidity (%)"=w565:sgl, "Acceleration vector (g)"=w564:sgl[])  [unwired: 10 in]
                  }
                }
                "Pressures" <- w522
                "Acceleration vector (g)" <- w518
                "Gyration vector (deg / s)" <- w517
                "Atmospheric pressure (mbar)" <- w514
                "External thermistor 0 temperature (deg C)" <- w516
                "Env. sensor die temperature (deg C)" <- w520
                "Relative humidity (%)" <- w519
                "External thermistor 1 temperature (deg C)" <- w515
                n160 = case shown="True" w526 {
                  tunnel: w499 -> [w575 w584]
                  tunnel: [w575 w584] -> w539
                  tunnel: w538 -> [_ w594]
                  tunnel: w524 -> [_ w582]
                  tunnel: w537 -> [w573 w591]
                  tunnel: w536 -> [w574 w590]
                  tunnel: [w574 w589] -> w535
                  tunnel: [w573 w588] -> w534
                  tunnel: w532 -> [w572 w583]
                  tunnel: [w572 w587] -> w533
                  tunnel: w531 -> [w571 w581]
                  tunnel: w530 -> [_ w580]
                  tunnel: [w571 w586] -> w529
                  tunnel: w528 -> [w570 w579]
                  tunnel: [w570 w585] -> w527
                  frame False {
                  }
                  frame True {
                    n161 = Add(x=w581, y=w580) -> (x+y=w576:sgl)
                    n162 = Build Array (concatenate)(w583, w582) -> (w577:sgl[][])
                    n163 = Build Array (concatenate)(w579, w581) -> (w578:sgl[])
                    n164 = Quotient & Remainder(x=w584, y=w594) -> (x-y*floor(x/y)=w593:u32)  [unwired: 1 out]
                    n165 = Equal To 0?(x=w593) -> (x = 0?=w592:bool)
                    n166 = case shown="True" w592 {
                      tunnel: w582 -> [_ _]
                      tunnel: w591 -> [w598 w612]
                      tunnel: w590 -> [w599 w611]
                      tunnel: [w599 w610] -> w589
                      tunnel: [w598 w609] -> w588
                      tunnel: w577 -> [w597 w604]
                      tunnel: [w597 sgl[][] []] -> w587
                      tunnel: w576 -> [w596 w607]
                      tunnel: [w596 w607] -> w586
                      tunnel: w578 -> [w595 w606]
                      tunnel: [w595 sgl[] []] -> w585
                      frame False {
                      }
                      frame True {
                        # "Write to disk every f samples (i.e. 1 s intervals)"
                        n167 = To Single Precision Float(number=w606) -> (single precision float=w600:sgl[])
                        n168 = Transpose 2D Array(2D array=w604) -> (transposed array=w603:sgl[][])
                        n169 = Build Array (concatenate)(w600, w603) -> (w602:sgl[][])
                        n170 = Transpose 2D Array(2D array=w602) -> (transposed array=w601:sgl[][])
                        n171 = Array To Spreadsheet String(delimiter (Tab)="\t", array=w601, 3:"%.4f" ("format string")) -> (spreadsheet string=w615:string)
                        n172 = Write to Text File(file (use dialog)=w612, text=w615, error in=w611) -> (refnum out=w609:refnum<file>, error out=w610:errorcluster)  [unwired: 1 in, 1 out]
                      }
                    }
                  }
                }
                n173 = local write "Checksum ok"(w501) -> ()
                n174 = Index Array(array=w522, index (row)=0) -> (element=w525:sgl[])  [unwired: 1 in]
              }
            }
            "chk err" <- w442
            "frm err" <- w443
            n175 = Equal?(x=w445, y=w447) -> (x = y?=w446:bool)
            n176 = call <vilib>:"Clear Errors.vi"("error in (no error)"=w460, "specific error code to clear (0: all)"=1073676294) -> ("error out"=w459:errorcluster)  [unwired: 4 in, 1 out]
            n177 = local write "Error"(w459) -> ()
            n178 = Compound Arithmetic op=OR(w459, "Stop Data", w446) -> (w477:bool)
          }
          n179 = case shown="True" w404 {
            tunnel: [w427 w441] -> w414
            tunnel: w409 -> [w427 w433]
            tunnel: w408 -> [_ w434]
            tunnel: w391 -> [_ w432]
            tunnel: w390 -> [_ w429]
            frame False {
            }
            frame True {
              # "Write any remaining data to disk, then close file"
              n180 = To Single Precision Float(number=w429) -> (single precision float=w428:sgl[])
              n181 = Transpose 2D Array(2D array=w432) -> (transposed array=w438:sgl[][])
              n182 = Build Array (concatenate)(w428, w438) -> (w439:sgl[][])
              n183 = Transpose 2D Array(2D array=w439) -> (transposed array=w440:sgl[][])
              n184 = Array To Spreadsheet String(delimiter (Tab)="\t", array=w440, 3:"%.4f" ("format string")) -> (spreadsheet string=w435:string)
              n185 = Write to Text File(file (use dialog)=w434, text=w435, error in=w433) -> (refnum out=w431:refnum<file>, error out=w430:errorcluster)  [unwired: 1 in, 1 out]
              n186 = Close File(refnum=w431, error in=w430) -> (error out=w441:errorcluster)  [unwired: 1 out]
            }
          }
          n187 = Transpose 2D Array(2D array=w383) -> (transposed array=w385:sgl[][])
          n188 = Transpose 2D Array(2D array=w377) -> (transposed array=w386:sgl[][])
          n189 = Transpose 2D Array(2D array=w378) -> (transposed array=w387:sgl[][])
          n190 = Multiply(x=w394, y=sgl 2000.0) -> (x*y=w395:sgl)
          n191 = To Unsigned Long Integer(number=w395) -> (unsigned 32bit integer=w392:u32)
          n192 = Build Array (concatenate)(w385, w382, w381, w380, w379, w376, w386, w387) -> (w384:sgl[][])
          n193 = call "8HP_Send Cmd.vi"("Operation"=T2 "d" ("Combo Box"), "Port"=w401) -> ("Error Out"=w398:errorcluster, "Port out"=w399:refnum<visa-resource-name>)  [unwired: 2 in]
          n194 = call "8HP_Clear buffer.vi"("Error in"=w398, "dt for timeout (ms)"=w392, "VISA resource name in"=w399) -> ("Error out"=w396:errorcluster, "VISA resource name out"=w397:refnum<visa-resource-name>)  [unwired: 3 in]
          n195 = call "8HP_Close serial port.vi"("Error in"=w396, "VISA resource name"=w397) -> ("Error out"=w415:errorcluster)  [unwired: 9 in]
        }
      }
      n196 = local write "Stream enabled"(w304) -> ()
      n197 = Merge Errors(w300, w301, w299) -> (w298:errorcluster)
    }
    frame "d" {
      # "Disable USB streaming"
      n198 = flat-sequence {
        tunnel: [w630] -> w623
        tunnel: w622 -> [w630]
        tunnel: w616 -> [w629]
        tunnel: [w624] -> w617
        tunnel: w623 -> [w639]
        tunnel: [w638] -> w621
        tunnel: [TRUE] -> w618
        tunnel: w617 -> [w632]
        frame #0 {
          n199 = Reciprocal(x=w629) -> (1/x=w628:dbl)
          n200 = disable-structure shown="Disabled" {
            frame Disabled {
              n201 = local write "Main"(T1."Data stream" ("Main")) -> ()
            }
            frame Enabled {
            }
          }
          n202 = To Single Precision Float(number=w628) -> (single precision float=w625:sgl)
          n203 = Multiply(x=w625, y=sgl 2000.0) -> (x*y=w626:sgl)
          n204 = To Unsigned Long Integer(number=w626) -> (unsigned 32bit integer=w624:u32)
        }
        frame #1 {
          n205 = local read "COM port"() -> (w640:refnum<visa-resource-name>)
          n206 = call "8HP_Open serial port.vi"("timeout (ms)"=u32 5000, "VISA resource name"=w640) -> ("Error out"=w641:errorcluster, "VISA resource name out"=w642:refnum<visa-resource-name>)  [unwired: 8 in]
          n207 = call "8HP_Send Cmd.vi"("Error In"=w641, "Operation"=w639, "Port"=w642) -> ("Error Out"=w636:errorcluster, "Port out"=w634:refnum<visa-resource-name>)  [unwired: 1 in]
          n208 = call "8HP_Clear buffer.vi"("Error in"=w636, "dt for timeout (ms)"=w632, "VISA resource name in"=w634) -> ("Error out"=w635:errorcluster, "VISA resource name out"=w633:refnum<visa-resource-name>)  [unwired: 3 in]
          n209 = call "8HP_Close serial port.vi"("Error in"=w635, "VISA resource name"=w633) -> ("Error out"=w638:errorcluster)  [unwired: 9 in]
        }
      }
    }
    frame "F" {
      # "Set data rate"
      n210 = flat-sequence {
        tunnel: w652 -> [w655]
        tunnel: [w655] -> w651
        tunnel: w651 -> [w662]
        tunnel: [w661] -> w650
        tunnel: [w660] -> w649
        tunnel: [w725] -> w648
        tunnel: w650 -> [w725]
        tunnel: w649 -> [w723]
        tunnel: [w723] -> w645
        tunnel: [TRUE] -> w644
        frame #0 {
          n211 = local write "Returned data rate (Hz)"(u16 0 ("Returned data rate (Hz)")) -> ()
          n212 = local write "received"(FALSE ("sent")) -> ()
          n213 = local write "Main"(T1."Data rate" ("Main")) -> ()
          n214 = local write "sent"(FALSE ("sent")) -> ()
        }
        frame #1 {
          # "to LE"
          n215 = local read "Set data rate (Hz)"() -> (w658:u8)
          n216 = case shown="14, Default" w658 {
            tunnel: [1.0 2.0 4.0 5.0 8.0 10.0 16.0 20.0 25.0 32.0 40.0 50.0 64.0 80.0 100.0 125.0 160.0 200.0 250.0 320.0 400.0 500.0 625.0 800.0 1000.0] -> w661
            tunnel: [u8 0 u8 0 u8 0 u8 0 u8 0 u8 0 u8 0 u8 0 u8 1 u8 1 u8 1 u8 2 u8 2 u8 2 u8 3 u8 3 u8 3 u8 4 u8 4 u8 4 u8 5 u8 5 u8 6 u8 6 u8 6] -> _
            frame 0 {
            }
            frame 1 {
            }
            frame 2 {
            }
            frame 3 {
            }
            frame 4 {
            }
            frame 5 {
            }
            frame 6 {
            }
            frame 7 {
            }
            frame 8 {
            }
            frame 9 {
            }
            frame 10 {
            }
            frame 11 {
            }
            frame 12 {
            }
            frame 13 {
            }
            frame 14, Default {
            }
            frame 15 {
            }
            frame 16 {
            }
            frame 17 {
            }
            frame 18 {
            }
            frame 19 {
            }
            frame 20 {
            }
            frame 21 {
            }
            frame 22 {
            }
            frame 23 {
            }
            frame 24 {
            }
          }
          n217 = local read "COM port"() -> (w665:refnum<visa-resource-name>)
          n218 = To Unsigned Word Integer(number=w661) -> (unsigned 16bit integer=w669:u16)
          n219 = Type Cast(type="", x=w669) -> (*(type *) &x=w671:string)
          n220 = call "8HP_Open serial port.vi"("timeout (ms)"=u32 5000, "VISA resource name"=w665) -> ("Error out"=w666:errorcluster, "VISA resource name out"=w667:refnum<visa-resource-name>)  [unwired: 8 in]
          n221 = Reverse String(1:w671) -> (0:w659:string)
          n222 = call "8HP_Send Cmd + Data.vi"("Error In"=w666, "Data"=w659, "Operation"=w662, "Port"=w667) -> ("Error Out"=w663:errorcluster, "Port out"=w664:refnum<visa-resource-name>)  [unwired: 1 in]
          n223 = call "8HP_Close serial port.vi"("Error in"=w663, "VISA resource name"=w664) -> ("Error out"=w660:errorcluster)  [unwired: 9 in]
        }
        frame #2 {
          n224 = Unbundle By Name(w723) -> ("status"=w724:bool)
          n225 = Not(x=w724) -> (.not. x?=→"sent":bool)
        }
      }
    }
    frame "f" {
      # "Get data rate"
      n226 = flat-sequence {
        tunnel: w735 -> [w738]
        tunnel: [w738] -> w734
        tunnel: w734 -> [w748]
        tunnel: [w751] -> w733
        tunnel: [w753] -> w732
        tunnel: [w760] -> w731
        tunnel: w733 -> [w760]
        tunnel: w732 -> [w758]
        tunnel: [w758] -> w728
        tunnel: [TRUE] -> w727
        frame #0 {
          n227 = local write "received"(FALSE ("sent")) -> ()
          n228 = local write "Main"(T1."Data rate" ("Main")) -> ()
          n229 = local write "sent"(FALSE ("sent")) -> ()
        }
        frame #1 {
          # "to BE"
          n230 = local read "COM port"() -> (w754:refnum<visa-resource-name>)
          n231 = call "8HP_Open serial port.vi"("timeout (ms)"=u32 5000, "VISA resource name"=w754) -> ("Error out"=w749:errorcluster, "VISA resource name out"=w750:refnum<visa-resource-name>)  [unwired: 8 in]
          n232 = call "8HP_Send Cmd.vi"("Error In"=w749, "Operation"=w748, "Port"=w750) -> ("Error Out"=w746:errorcluster, "Port out"=w745:refnum<visa-resource-name>)  [unwired: 1 in]
          n233 = VISA Read(VISA resource name=w745, byte count=u32 2, error in (no error)=w746) -> (VISA resource name out=w743:refnum<visa-resource-name>, read buffer=w742:string, error out=w744:errorcluster)  [unwired: 1 out]
          n234 = Reverse String(1:w742) -> (0:w752:string)
          n235 = call "8HP_Close serial port.vi"("Error in"=w744, "VISA resource name"=w743) -> ("Error out"=w753:errorcluster)  [unwired: 9 in]
          n236 = Type Cast(type=u16 0 ("byte count"), x=w752) -> (*(type *) &x=w740:u16)
          "Returned data rate (Hz)" <- w740
          n237 = To Double Precision Float(number=w740) -> (double precision float=w751:dbl)
        }
        frame #2 {
          n238 = Unbundle By Name(w758) -> ("status"=w759:bool)
          n239 = Not(x=w759) -> (.not. x?=→"received":bool)
        }
      }
    }
    frame "N" {
      # "Get serial number"
      n240 = flat-sequence {
        tunnel: w764 -> [w770]
        tunnel: [w770] -> w763
        tunnel: [TRUE] -> w767
        tunnel: w763 -> [w776]
        tunnel: [w775] -> w762
        frame #0 {
          n241 = local write "Main"(T1."Action" ("Main")) -> ()
          "Serial number" <- sgl 0.0 ("Numeric")
        }
        frame #1 {
          # "to BE"
          n242 = local read "COM port"() -> (w777:refnum<visa-resource-name>)
          n243 = call "8HP_Open serial port.vi"("timeout (ms)"=u32 5000, "VISA resource name"=w777) -> ("Error out"=w784:errorcluster, "VISA resource name out"=w785:refnum<visa-resource-name>)  [unwired: 8 in]
          n244 = call "8HP_Send Cmd.vi"("Error In"=w784, "Operation"=w776, "Port"=w785) -> ("Error Out"=w782:errorcluster, "Port out"=w783:refnum<visa-resource-name>)  [unwired: 1 in]
          n245 = VISA Read(VISA resource name=w783, byte count=u32 4, error in (no error)=w782) -> (VISA resource name out=w780:refnum<visa-resource-name>, read buffer=w772:string, error out=w779:errorcluster)  [unwired: 1 out]
          n246 = call "8HP_Close serial port.vi"("Error in"=w779, "VISA resource name"=w780) -> ("Error out"=w775:errorcluster)  [unwired: 9 in]
          n247 = Reverse String(1:w772) -> (0:w773:string)
          n248 = Type Cast(type=sgl 0.0 ("byte count"), x=w773) -> (*(type *) &x=w771:sgl)
          n249 = local write "Serial number"(w771) -> ()
        }
      }
    }
    frame "X" {
      # "Exit"
    }
    frame Default {
    }
  }
  "All samples out" <- w2
  n250 = Merge Errors(w11, w10, w9) -> (w8:errorcluster)
  n251 = call <vilib>:"Clear Errors.vi"("error in (no error)"=w8, "specific error code to clear (0: all)"=1073676294) -> ("error out"=w5:errorcluster)  [unwired: 4 in, 1 out]
  n252 = local write "Error"(w5) -> ()
  n253 = Release Queue(queue=w6, error in (no error)=w5) -> (error out=→"Error":errorcluster)  [unwired: 1 in, 2 out]
